vi "Arduino Stepper Driver XY subVI queryPosition.vi"(8 "error in (no error)":errorcluster, 11 "VISA resource name":refnum<visa-resource-name>) -> (0 "error out":errorcluster, 1 "Vertical driver position":i32, 2 "Horizontal driver position":i32, 3 "VISA resource name out":refnum<visa-resource-name>)   [LabVIEW 2013]
panel:
  out "read buffer":string
  out "return count":u32
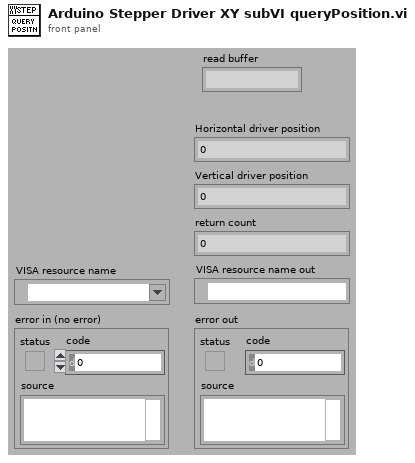
[diagram p1: front panel]
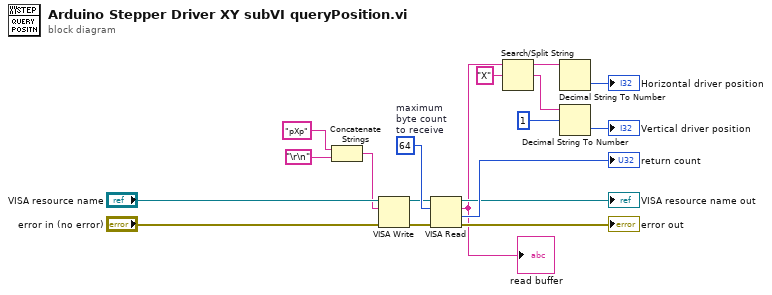
[diagram p0: block diagram]
diagram:
  w12 = u32 64  # maximum byte count to receive
  n1 = Concatenate Strings("pXp" ("string"), "\r\n") -> (w10:string)
  n2 = VISA Write(VISA resource name="VISA resource name", write buffer=w10, error in (no error)="error in (no error)") -> (VISA resource name out=w9:refnum<visa-resource-name>, error out=w8:errorcluster)  [unwired: 1 out]
  n3 = VISA Read(VISA resource name=w9, byte count=w12, error in (no error)=w8) -> (VISA resource name out=→"VISA resource name out":refnum<visa-resource-name>, read buffer=w5:string, return count=→"return count":u32, error out=→"error out":errorcluster)
  "read buffer" <- w5
  n4 = Search/Split String(string=w5, search string/char (-)="X") -> (substring before match=w3:string, match + rest of string=w1:string)  [unwired: 1 in, 1 out]
  n5 = Decimal String To Number(string=w3) -> (number=→"Horizontal driver position":i32)  [unwired: 2 in, 1 out]
  n6 = Decimal String To Number(string=w1, offset=1 ("offset (0)")) -> (number=→"Vertical driver position":i32)  [unwired: 1 in, 1 out]
